vi "GEOM_GetTopo_1readmode.vi"(9 "GEOM_FPAReadModes":T1[](array[typedef]) {"Amplifiers"."fliped" items=["none", "horizontal", "vertical"]; "Amplifiers"."type" items=["LL", "LR", "UL", "UR"]}, 10 "readmode":string) -> (2 "strinfo":string)   [LabVIEW 2016]
uses:
  GEOM_FPAReadMode.ctl
  GEOM_Amplifier.ctl
  GEOM_AmpType.ctl
  GEOM_ROI.ctl
  GEOM_Coords.ctl
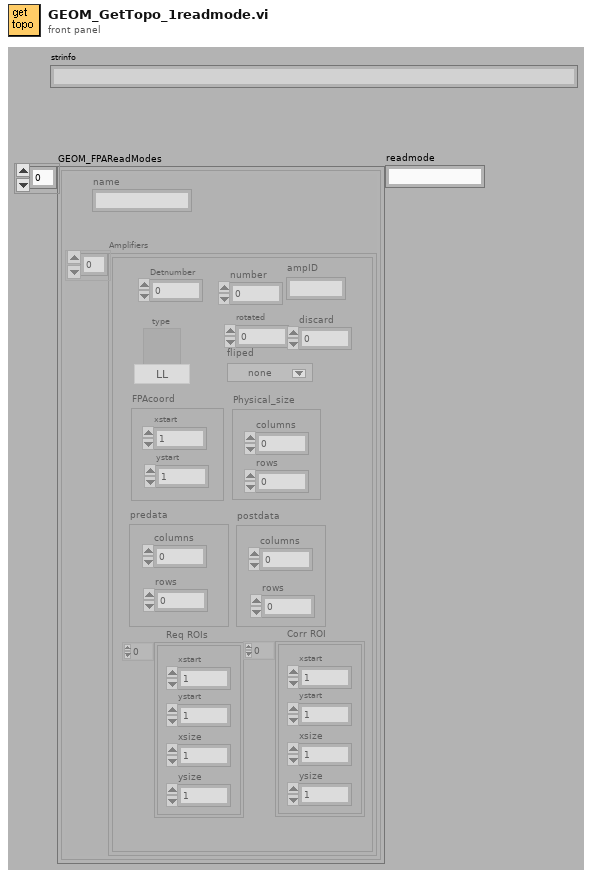
[diagram p1: front panel]
types:
  T1 = typedef "GEOM_FPAReadMode.ctl" = cluster{"name":string, "Amplifiers":T2[]}
  T2 = typedef "GEOM_Amplifier.ctl" = cluster{"number":i32, "type":T3, "rotated":i16, "fliped":u16, "FPAcoord":cluster{"xstart":i32, "ystart":i32}, "Physical_size":cluster{"columns":i32, "rows":i32}, "predata":cluster{"columns":i32, "rows":i32}, "postdata":cluster{"columns":i32, "rows":i32}, "Req ROIs":T4, "Corr ROI":T4, "Detnumber":i32, "ampID":string, "discard":i32}
  T3 = typedef "GEOM_AmpType.ctl" = u16
  T4 = typedef "GEOM_ROI.ctl" = T5[]
  T5 = typedef "GEOM_Coords.ctl" = cluster{"xstart":u32, "ystart":u32, "xsize":u32, "ysize":u32}
  T6 = typedef "GEOM_CorrectedFPA.ctl" = cluster{"readmode":string, "amplifiers":cluster{"number":i32, "xstart":i32, "ystart":i32}[], "totxsize":i32, "totysize":i32, "maxxdim":i32, "maxydim":i32, "numxamps":i32, "numyamps":i32, "totxdata":i32, "totydata":i32, "xdataamp":i32, "ydataamp":i32, "totpixels":i32}
  T7 = cluster{"number":i32, "xstart":i32, "ystart":i32}[]
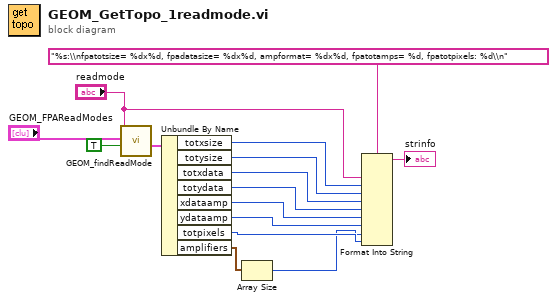
[diagram p0: block diagram]
diagram:
  n1 = call "GEOM_findReadMode.vi"("binning corrected?"=TRUE, "GEOM_FPAReadModes"="GEOM_FPAReadModes", "readmode"="readmode") -> ("BinFPA"=w14:T6)  [unwired: 8 out]
  n2 = Unbundle By Name(w14) -> ("totxsize"=w9:i32, "totysize"=w8:i32, "totxdata"=w7:i32, "totydata"=w6:i32, "xdataamp"=w5:i32, "ydataamp"=w4:i32, "totpixels"=w2:i32, "amplifiers"=w11:T7)
  n3 = Array Size(array=w11) -> (size(s)=w1:i32)
  n4 = Format Into String(format string="%s:\\nfpatotsize= %dx%d, fpadatasize= %dx%d, ampformat= %dx%d, fpatotamps= %d, fpatotpixels: %d\\n", "readmode", w9, w8, w7, w6, w5, w4, w1, w2) -> (resulting string=→"strinfo":string)  [unwired: 2 in, 1 out]
